vi "[Global] CameraNameArray.vi"() -> ()   [LabVIEW 2019]
panel:
  in  "CameraNameArray":string[](array[string])
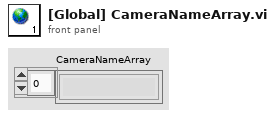
[diagram p1: front panel]
diagram:
